vi "Get cif_manager_RegisterPluginLoaderRequest.vi"(8 "error in (no error)":errorcluster, 11 "gRPCid":T1) -> (0 "error out":errorcluster, 2 "package_templatemessage":T2, 3 "gRPCid out":T1)   [LabVIEW 2021, in "CIF_Manager_server.lvlib"]
uses:
  CIF_Manager_server.lvlib
  cif_manager_RegisterPluginLoaderRequest.ctl
  cif_manager_LoaderInfoFull.ctl
  cif_manager_LoaderType.ctl
  <vilib>/gRPC/LabVIEW gRPC Library/Shared/grpcId.ctl
  cif_manager_RegisterPluginLoaderRequest_Flat.ctl
  cif_manager_LoaderInfoFull_Flat.ctl
  2ed25e12-861d-4677-8ead-ace2906b2041.vi
  <vilib>/gRPC/LabVIEW gRPC Library/Shared/TranslateGrpcError.vi
  FlatToRichcif_manager_LoaderInfoFull.vi
  <vilib>/gRPC/LabVIEW gRPC Library/Server API/Server/Get Server DLL Path.vi
  <vilib>/Utility/error.llb/Error Cluster From Error Code.vi
  <vilib>/gRPC/LabVIEW gRPC Library/grpc-lvsupport-release.lvlib
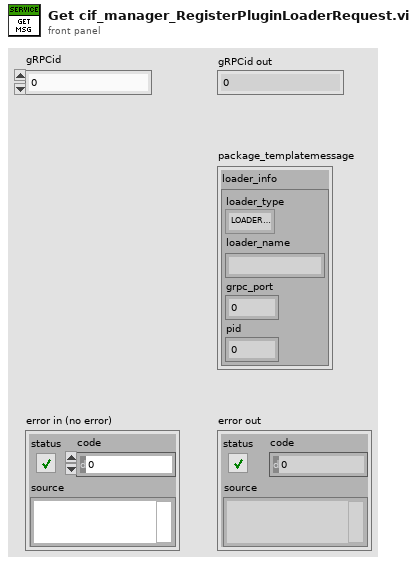
[diagram p1: front panel]
types:
  T1 = typedef "grpc-lvsupport-release.lvlib/grpcId.ctl" = u64
  T2 = typedef "CIF_Manager_server.lvlib/cif_manager_RegisterPluginLoaderRequest.ctl" = cluster{"loader_info":T3}
  T3 = typedef "CIF_Manager_server.lvlib/cif_manager_LoaderInfoFull.ctl" = cluster{"loader_type":T4, "loader_name":string, "grpc_port":i32, "pid":u32}
  T4 = typedef "CIF_Manager_server.lvlib/cif_manager_LoaderType.ctl" = enum32{"LOADERTYPE_UNKNOWN", "LOADERTYPE_LABVIEW"}
  T5 = typedef "CIF_Manager_server.lvlib/cif_manager_RegisterPluginLoaderRequest_Flat.ctl" = cluster{"loader_info":T6}
  T6 = typedef "CIF_Manager_server.lvlib/cif_manager_LoaderInfoFull_Flat.ctl" = cluster{"loader_type":T4, "loader_name":string, "grpc_port":i32, "pid":u32}
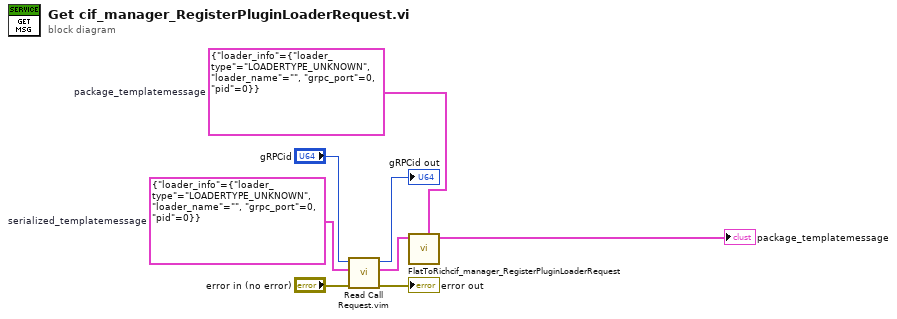
[diagram p0: block diagram]
diagram:
  w6 = T5 {"loader_info"={"loader_type"=enum."LOADERTYPE_UNKNOWN", "loader_name"="", "grpc_port"=0, "pid"=0}}  # serialized_templatemessage
  w5 = T2 {"loader_info"={"loader_type"=enum."LOADERTYPE_UNKNOWN", "loader_name"="", "grpc_port"=0, "pid"=0}}  # package_templatemessage
  n1 = call "Read Call Request.vim"("error in"="error in (no error)", "Request Type"=w6, "gRPCid in"="gRPCid") -> ("error out"=→"error out":errorcluster, "Request Data"=w4:T5, "gRPCid out"=→"gRPCid out":T1)  [unwired: 6 in]
  n2 = call "FlatToRichcif_manager_RegisterPluginLoaderRequest.vi"("OutputClusterType"=w5, "InputCluster"=w4) -> ("OutputCluster"=→"package_templatemessage":T2)  [unwired: 9 in]
